vi "Build Setup Arrays.vi"(0 "Preview In":T1 {"Field" format="%.2f"}, 1 "Measure ?":bool, 2 "First Field":dbl format="%.2f", 3 "N Points":i32, 11 "error in (no error)":errorcluster, 12 "Last Field":dbl format="%.2f", 13 "Direction":bool, 14 "Average During Loop ?":bool) -> (4 "Preview Out":T1 {"Field" format="%.2f"}, 15 "error out":errorcluster)   [LabVIEW 2012, in "Multi Segment Waveform.xctl"]
doc: "Builds the arrays used to work out which data storage location each point should go in, assuming it is to be stored at all."
uses:
  Multi Segment Waveform.xctl
  <vilib>/Analysis/1siggen.llb/Ramp Pattern by Samples.vi
  <vilib>/Analysis/NI_AALBase.lvlib
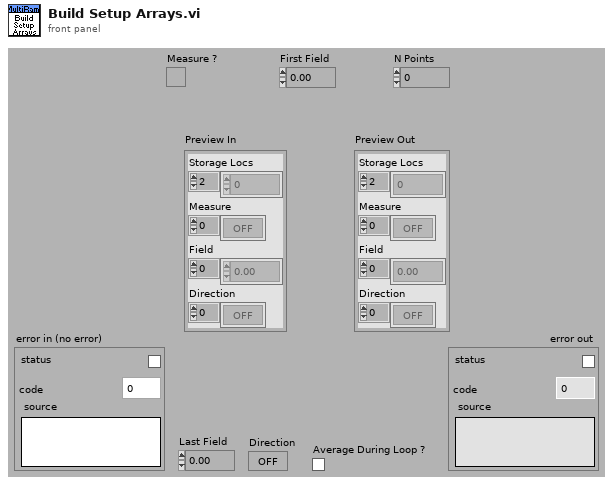
[diagram p1: front panel]
types:
  T1 = cluster{"Storage Locs":i32[], "Measure":bool[], "Field":dbl[], "Direction":bool[]}
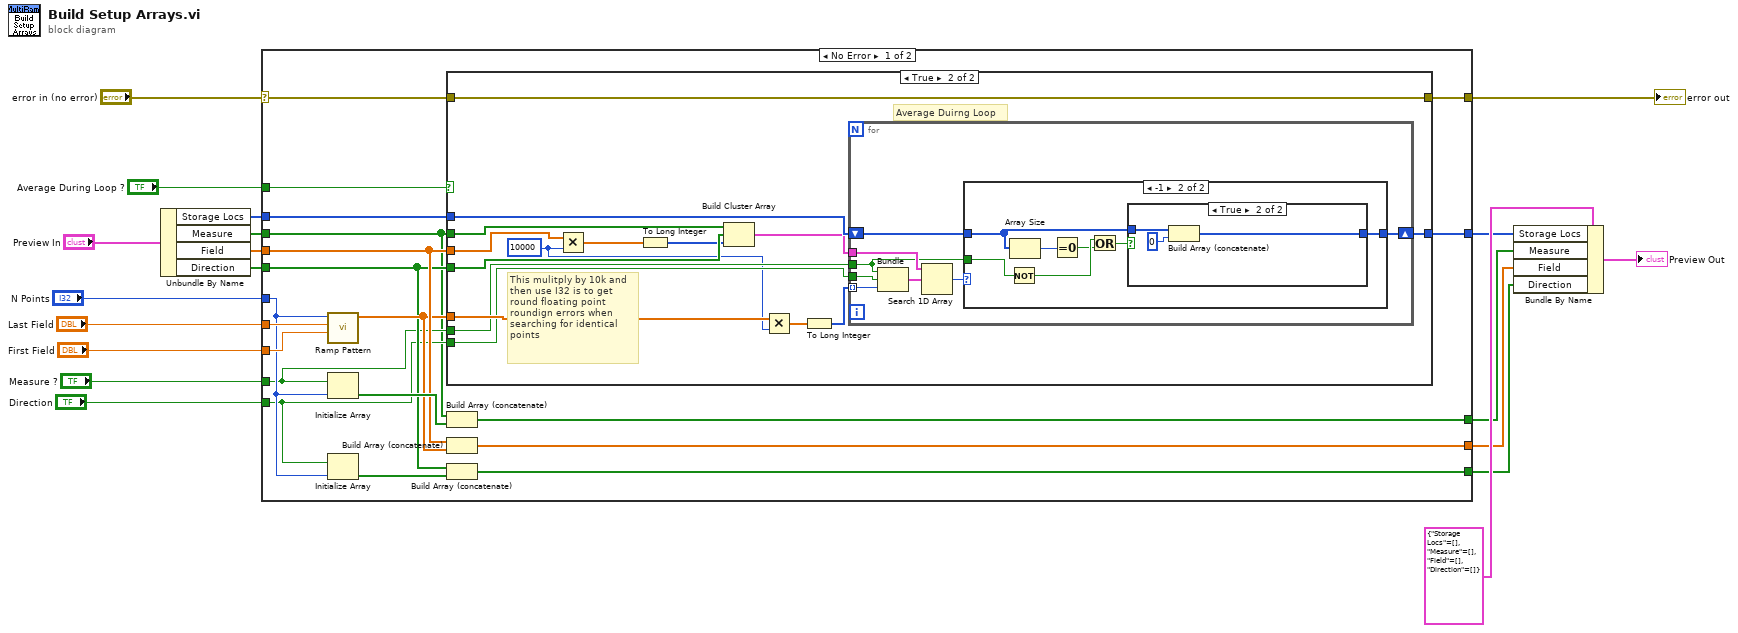
[diagram p0: block diagram]
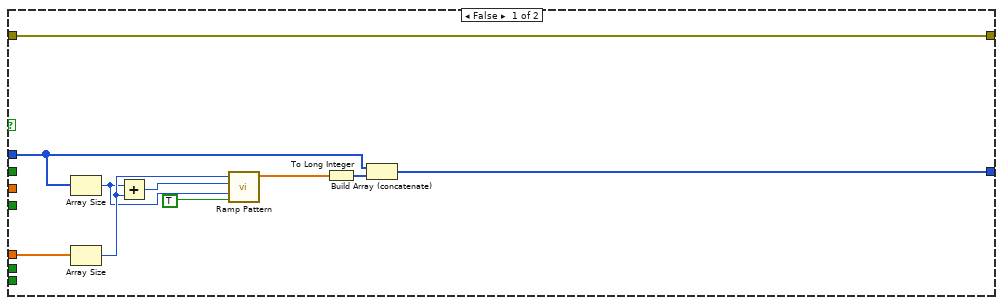
[diagram p2: hidden frame]
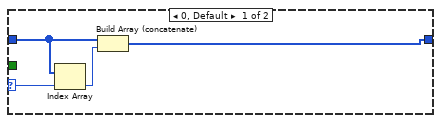
[diagram p3: hidden frame]
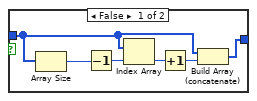
[diagram p4: hidden frame]
diagram:
  n1 = Unbundle By Name("Preview In") -> ("Storage Locs"=w10:i32[], "Measure"=w9:bool[], "Field"=w7:dbl[], "Direction"=w8:bool[])
  n2 = case shown="No Error" "error in (no error)" {
    selector: "error in (no error)" -> [w21 w92]
    tunnel: "First Field" -> [w38 _]
    tunnel: "Last Field" -> [w37 _]
    tunnel: "N Points" -> [w36 _]
    tunnel: w7 -> [w33 _]
    tunnel: [w32 _] -> w3
    tunnel: [w31 _] -> w4
    tunnel: [w30 _] -> w2
    tunnel: "Average During Loop ?" -> [w29 _]
    tunnel: w8 -> [w27 _]
    tunnel: w10 -> [w26 _]
    tunnel: "Direction" -> [w25 _]
    tunnel: [w24 _] -> w1
    tunnel: "Measure ?" -> [w23 _]
    tunnel: w9 -> [w22 _]
    tunnel: [w20 w92] -> w12
    frame No Error {
      n3 = call-poly <vilib>:"Ramp Pattern.vi"("start"=w38, "end"=w37, "samples"=w36) -> ("Ramp Pattern"=w28:dbl[])  [unwired: 7 in, 1 out]
      n4 = Initialize Array(w23, w36) -> (w35:bool[])
      n5 = Initialize Array(w25, w36) -> (w34:bool[])
      n6 = case shown="True" w29 {
        tunnel: w33 -> [_ w54]
        tunnel: w28 -> [w46 w61]
        tunnel: w27 -> [_ w62]
        tunnel: w26 -> [w45 w63]
        tunnel: w25 -> [_ w60]
        tunnel: [w47 w58] -> w24
        tunnel: w23 -> [_ w57]
        tunnel: w22 -> [_ w56]
        tunnel: w21 -> [w39 w49]
        tunnel: [w39 w49] -> w20
        frame False {
          n7 = Array Size(array=w45) -> (size(s)=w42:i32)
          n8 = Array Size(array=w46) -> (size(s)=w43:i32)
          n9 = Add(x=w42, y=w43) -> (x+y=w41:i32)
          n10 = call-poly <vilib>:"Ramp Pattern.vi"("exclude end?"=TRUE, "start"=w42, "end"=w41, "samples"=w43) -> ("Ramp Pattern"=w48:dbl[])  [unwired: 6 in, 1 out]
          n11 = To Long Integer(number=w48) -> (32bit integer=w44:i32[])
          n12 = Build Array (concatenate)(w45, w44) -> (w47:i32[])
        }
        frame True {
          w51 = 10000
          # "This mulitply by 10k and\nthen use I32 is to get\nround floating point\nroundign errors when\nsearching for identical\npoints"
          # "Average Duirng Loop"
          n13 = Multiply(x=w54, y=w51) -> (x*y=w55:dbl[])
          n14 = To Long Integer(number=w55) -> (32bit integer=w53:i32[])
          n15 = Build Cluster Array(w56, w62, w53) -> (w59:cluster{bool, bool, i32}[])
          n16 = Multiply(x=w61, y=w51) -> (x*y=w52:dbl[])
          n17 = To Long Integer(number=w52) -> (32bit integer=w50:i32[])
          n18 = for {
            tunnel: w50 -> [w70] mode=indexing
            shift-right: [w67] -> w58
            shift-left: w63 -> [w68]
            tunnel: w60 -> [w71]
            tunnel: w59 -> [w66]
            tunnel: w57 -> [w64]
            n19 = Bundle("Measure ?"=w64, "Direction"=w71, w70) -> (w65:cluster{"Measure ?":bool, "Direction":bool, i32})  [unwired: 1 out]
            n20 = Search 1D Array(1D array=w66, element=w65) -> (index of element=w69:i32)  [unwired: 1 out]
            n21 = case shown="-1" w69 {
              selector: w69 -> [w75 _]
              tunnel: w68 -> [w73 w78]
              tunnel: [w72 w82] -> w67
              tunnel: w64 -> [_ w81]
              frame 0, Default {
                n22 = Index Array(array=w73, index=w75) -> (element=w74:i32)
                n23 = Build Array (concatenate)(w73, w74) -> (w72:i32[])
              }
              frame -1 {
                n24 = Not(x=w81) -> (.not. x?=w80:bool)
                n25 = Array Size(array=w78) -> (size(s)=w77:i32)
                n26 = Equal To 0?(x=w77) -> (x = 0?=w76:bool)
                n27 = Or(x=w80, y=w76) -> (x .or. y?=w79:bool)
                n28 = case shown="True" w79 {
                  tunnel: w78 -> [w84 w91]
                  tunnel: [w83 w90] -> w82
                  frame False {
                    n29 = Array Size(array=w84) -> (size(s)=w88:i32)
                    n30 = Decrement(x=w88) -> (x-1=w87:i32)
                    n31 = Index Array(array=w84, index=w87) -> (element=w86:i32)
                    n32 = Increment(x=w86) -> (x+1=w85:i32)
                    n33 = Build Array (concatenate)(w84, w85) -> (w83:i32[])
                  }
                  frame True {
                    n34 = Build Array (concatenate)(w91, 0 ("Input Element")) -> (w90:i32[])
                  }
                }
              }
            }
          }
        }
      }
      n35 = Build Array (concatenate)(w22, w35) -> (w30:bool[])
      n36 = Build Array (concatenate)(w33, w28) -> (w32:dbl[])
      n37 = Build Array (concatenate)(w27, w34) -> (w31:bool[])
    }
    frame Error {
    }
  }
  "error out" <- w12
  n38 = Bundle By Name(cluster=T1 {"Storage Locs"=[], "Measure"=[], "Field"=[], "Direction"=[]} ("Preview Out"), "Storage Locs"=w1, "Measure"=w2, "Field"=w3, "Direction"=w4) -> (→"Preview Out":T1)
